vi "Cut out additional spaces.vi"(2 "String":string, 3 "Mode":u16(ring) items=["All Spaces", "Only if 1st char.", "Only if last char.", "Only if near \"=\"", "Only if 1st or last char.", "Only multiple", "Really all"]) -> (14 "String out":string)   [LabVIEW 2020]
doc: "Searches for spaces in String and cuts them out if the following character is not LF."
panel:
  # "Searches for spaces in \"String\" and cuts them out, \ndepending on \"Mode\""
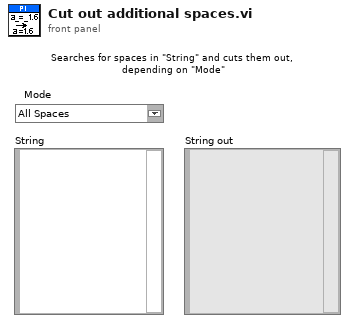
[diagram p1: front panel]
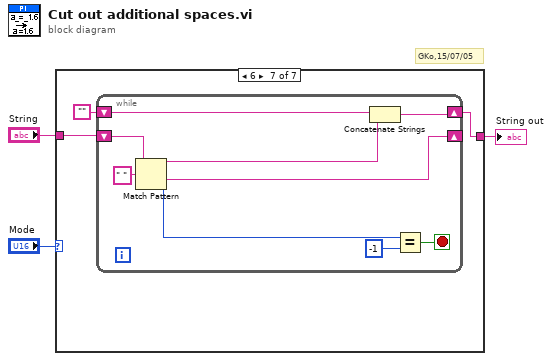
[diagram p0: block diagram]
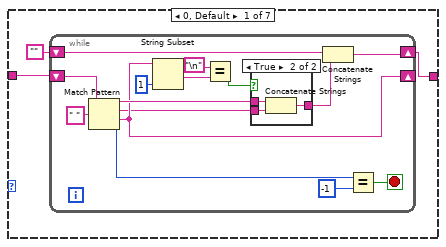
[diagram p2: hidden frame]
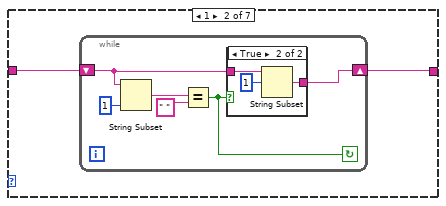
[diagram p4: hidden frame]
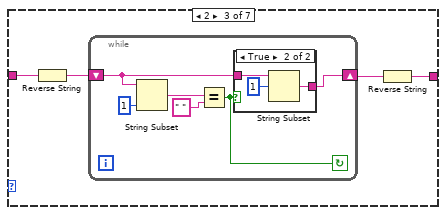
[diagram p6: hidden frame]
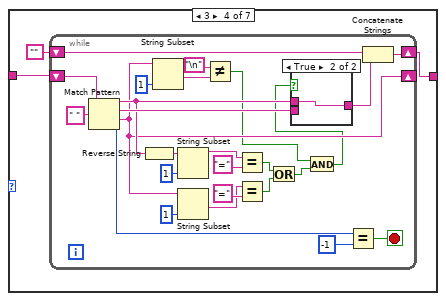
[diagram p8: hidden frame]
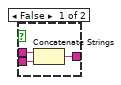
[diagram p9: hidden frame]
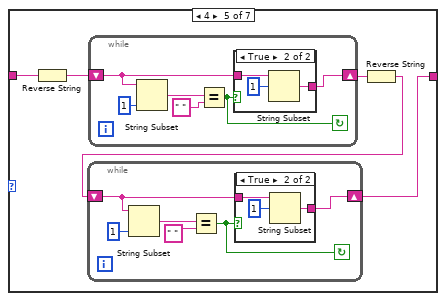
[diagram p10: hidden frame]
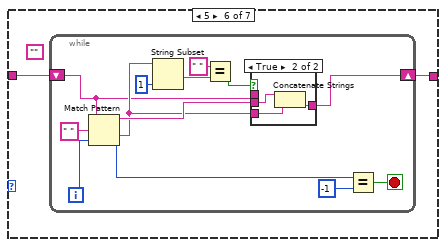
[diagram p13: hidden frame]
diagram:
  # "GKo,15/07/05"
  n1 = case shown="6" "Mode" {
    tunnel: "String" -> [w5 w27 w39 w53 w87 w111 w130]
    tunnel: [w4 w26 w38 w52 w85 w110 w129] -> w1
    frame 0, Default {
      n2 = while {
        shift-right: [w10] -> _
        shift-left: w5 -> [w7]
        shift-right: [w13] -> w4
        shift-left: "" -> [w12]
        stop <- w14 stop-if-true
        n3 = Match Pattern(string=w7, regular expression=" " ("search string")) -> (before substring=w16:string, match substring=w9:string, after substring=w10:string, offset past match=w8:i32)  [unwired: 1 out]
        n4 = String Subset(string=w10, length (rest)=1 ("length (rest)")) -> (substring=w19:string)  [unwired: 1 out]
        n5 = Equal?(x="\n", y=w19) -> (x = y?=w17:bool)
        n6 = case shown="True" w17 {
          tunnel: [w22 w25] -> w11
          tunnel: w16 -> [w22 w24]
          tunnel: w9 -> [_ w23]
          frame False {
          }
          frame True {
            n7 = Concatenate Strings(w24, w23) -> (w25:string)
          }
        }
        n8 = Concatenate Strings(w12, w11) -> (w13:string)
        n9 = Equal?(x=w8, y=-1) -> (x = y?=w14:bool)
      }
    }
    frame 1 {
      n10 = while {
        shift-right: [w29] -> w26
        shift-left: w27 -> [w30]
        stop <- w28 continue-if-true
        n11 = String Subset(string=w30, length (rest)=1 ("length (rest)")) -> (substring=w32:string)  [unwired: 1 out]
        n12 = Equal?(x=w32, y=" " ("search string")) -> (x = y?=w28:bool)
        n13 = case shown="True" w28 {
          tunnel: w30 -> [w34 w37]
          tunnel: [w34 w35] -> w29
          frame False {
          }
          frame True {
            n14 = String Subset(string=w37, offset (0)=1) -> (substring=w35:string)  [unwired: 1 out]
          }
        }
      }
    }
    frame 2 {
      n15 = Reverse String(1:w39) -> (0:w40:string)
      n16 = while {
        shift-right: [w44] -> w41
        shift-left: w40 -> [w43]
        stop <- w42 continue-if-true
        n17 = String Subset(string=w43, length (rest)=1 ("length (rest)")) -> (substring=w46:string)  [unwired: 1 out]
        n18 = Equal?(x=w46, y=" " ("search string")) -> (x = y?=w42:bool)
        n19 = case shown="True" w42 {
          tunnel: w43 -> [w48 w51]
          tunnel: [w48 w49] -> w44
          frame False {
          }
          frame True {
            n20 = String Subset(string=w51, offset (0)=1) -> (substring=w49:string)  [unwired: 1 out]
          }
        }
      }
      n21 = Reverse String(1:w41) -> (0:w38:string)
    }
    frame 3 {
      n22 = while {
        shift-right: [w58] -> _
        shift-left: w53 -> [w69]
        shift-right: [w74] -> w52
        shift-left: "" -> [w73]
        stop <- w75 stop-if-true
        n23 = Match Pattern(string=w69, regular expression=" " ("search string")) -> (before substring=w63:string, match substring=w71:string, after substring=w58:string, offset past match=w70:i32)  [unwired: 1 out]
        n24 = Reverse String(1:w63) -> (0:w62:string)
        n25 = String Subset(string=w58, length (rest)=1 ("length (rest)")) -> (substring=w78:string)  [unwired: 1 out]
        n26 = String Subset(string=w62, length (rest)=1 ("length (rest)")) -> (substring=w61:string)  [unwired: 1 out]
        n27 = String Subset(string=w58, length (rest)=1 ("length (rest)")) -> (substring=w59:string)  [unwired: 1 out]
        n28 = Not Equal?(x="\n", y=w78) -> (x != y?=w56:bool)
        n29 = Equal?(x=w61, y="=") -> (x = y?=w67:bool)
        n30 = Equal?(x=w59, y="=") -> (x = y?=w65:bool)
        n31 = Or(x=w67, y=w65) -> (x .or. y?=w57:bool)
        n32 = And(x=w56, y=w57) -> (x .and. y?=w55:bool)
        n33 = case shown="True" w55 {
          tunnel: [w83 w84] -> w72
          tunnel: w63 -> [w82 w84]
          tunnel: w71 -> [w81 _]
          frame False {
            n34 = Concatenate Strings(w82, w81) -> (w83:string)
          }
          frame True {
          }
        }
        n35 = Equal?(x=w70, y=-1) -> (x = y?=w75:bool)
        n36 = Concatenate Strings(w73, w72) -> (w74:string)
      }
    }
    frame 4 {
      n37 = Reverse String(1:w87) -> (0:w88:string)
      n38 = while {
        shift-right: [w102] -> w89
        shift-left: w88 -> [w101]
        stop <- w100 continue-if-true
        n39 = String Subset(string=w101, length (rest)=1 ("length (rest)")) -> (substring=w104:string)  [unwired: 1 out]
        n40 = Equal?(x=w104, y=" " ("search string")) -> (x = y?=w100:bool)
        n41 = case shown="True" w100 {
          tunnel: w101 -> [w106 w109]
          tunnel: [w106 w107] -> w102
          frame False {
          }
          frame True {
            n42 = String Subset(string=w109, offset (0)=1) -> (substring=w107:string)  [unwired: 1 out]
          }
        }
      }
      n43 = Reverse String(1:w89) -> (0:w86:string)
      n44 = while {
        shift-right: [w91] -> w85
        shift-left: w86 -> [w92]
        stop <- w90 continue-if-true
        n45 = String Subset(string=w92, length (rest)=1 ("length (rest)")) -> (substring=w94:string)  [unwired: 1 out]
        n46 = Equal?(x=w94, y=" " ("search string")) -> (x = y?=w90:bool)
        n47 = case shown="True" w90 {
          tunnel: w92 -> [w96 w99]
          tunnel: [w96 w97] -> w91
          frame False {
          }
          frame True {
            n48 = String Subset(string=w99, offset (0)=1) -> (substring=w97:string)  [unwired: 1 out]
          }
        }
      }
    }
    frame 5 {
      (unwired) ""
      n49 = while {
        shift-right: [w115] -> w110
        shift-left: w111 -> [w113]
        i -> [w116]
        stop <- w118 stop-if-true
        n50 = Match Pattern(string=w113, regular expression=" " ("search string"), offset (0)=w116) -> (before substring=w120:string, after substring=w114:string, offset past match=w117:i32)  [unwired: 1 out]
        n51 = String Subset(string=w114, length (rest)=1 ("length (rest)")) -> (substring=w122:string)  [unwired: 1 out]
        n52 = Equal?(x=" " ("search string"), y=w122) -> (x = y?=w121:bool)
        n53 = case shown="True" w121 {
          tunnel: [w125 w128] -> w115
          tunnel: w120 -> [_ w127]
          tunnel: w114 -> [_ w126]
          tunnel: w113 -> [w125 _]
          frame False {
          }
          frame True {
            n54 = Concatenate Strings(w127, w126) -> (w128:string)
          }
        }
        n55 = Equal?(x=w117, y=-1) -> (x = y?=w118:bool)
      }
    }
    frame 6 {
      n56 = while {
        shift-right: [w134] -> _
        shift-left: w130 -> [w132]
        shift-right: [w136] -> w129
        shift-left: "" -> [w135]
        stop <- w137 stop-if-true
        n57 = Match Pattern(string=w132, regular expression=" " ("search string")) -> (before substring=w139:string, after substring=w134:string, offset past match=w133:i32)  [unwired: 2 out]
        n58 = Concatenate Strings(w135, w139) -> (w136:string)
        n59 = Equal?(x=w133, y=-1) -> (x = y?=w137:bool)
      }
    }
  }
  "String out" <- w1
